vi "Read Steps From File - XML.vi"(11 "XML file path":path) -> (0 "error out":errorcluster, 3 "Sequence File Data":T1)   [LabVIEW 2011]
uses:
  HelperVIs.llb/SequenceFileData.ctl
  HelperVIs.llb/SequenceData.ctl
  HelperVIs.llb/StepGroup.ctl
  HelperVIs.llb/StepData.ctl
  HelperVIs.llb/StepProperties.ctl
  <vilib>/xml/Load XML File.vi
  <vilib>/xml/NI_XML.lvlib
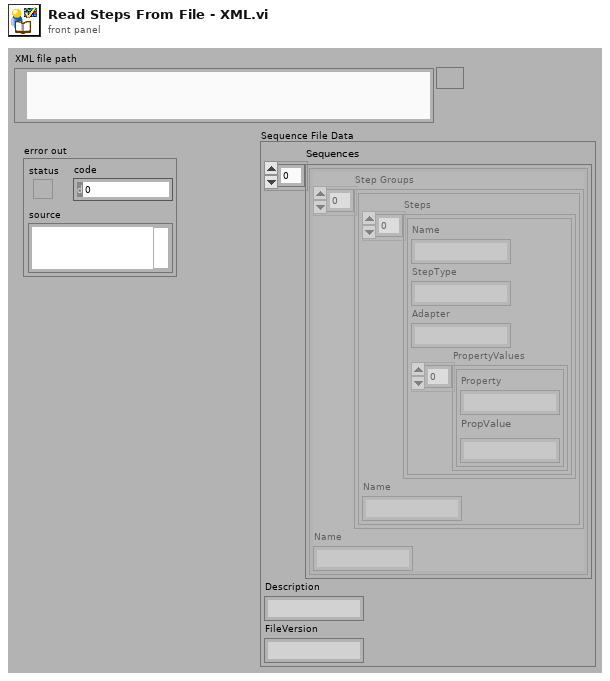
[diagram p1: front panel]
types:
  T1 = typedef "SequenceFileData.ctl" = cluster{"Sequences":T2[], "Description":string, "FileVersion":string}
  T2 = typedef "SequenceData.ctl" = cluster{"Step Groups":T3[], "Name":string}
  T3 = typedef "StepGroup.ctl" = cluster{"Steps":T4[], "Name":string}
  T4 = typedef "StepData.ctl" = cluster{"Name":string, "StepType":string, "Adapter":string, "PropertyValues":T5[]}
  T5 = typedef "StepProperties.ctl" = cluster{"Property":string, "PropValue":string}
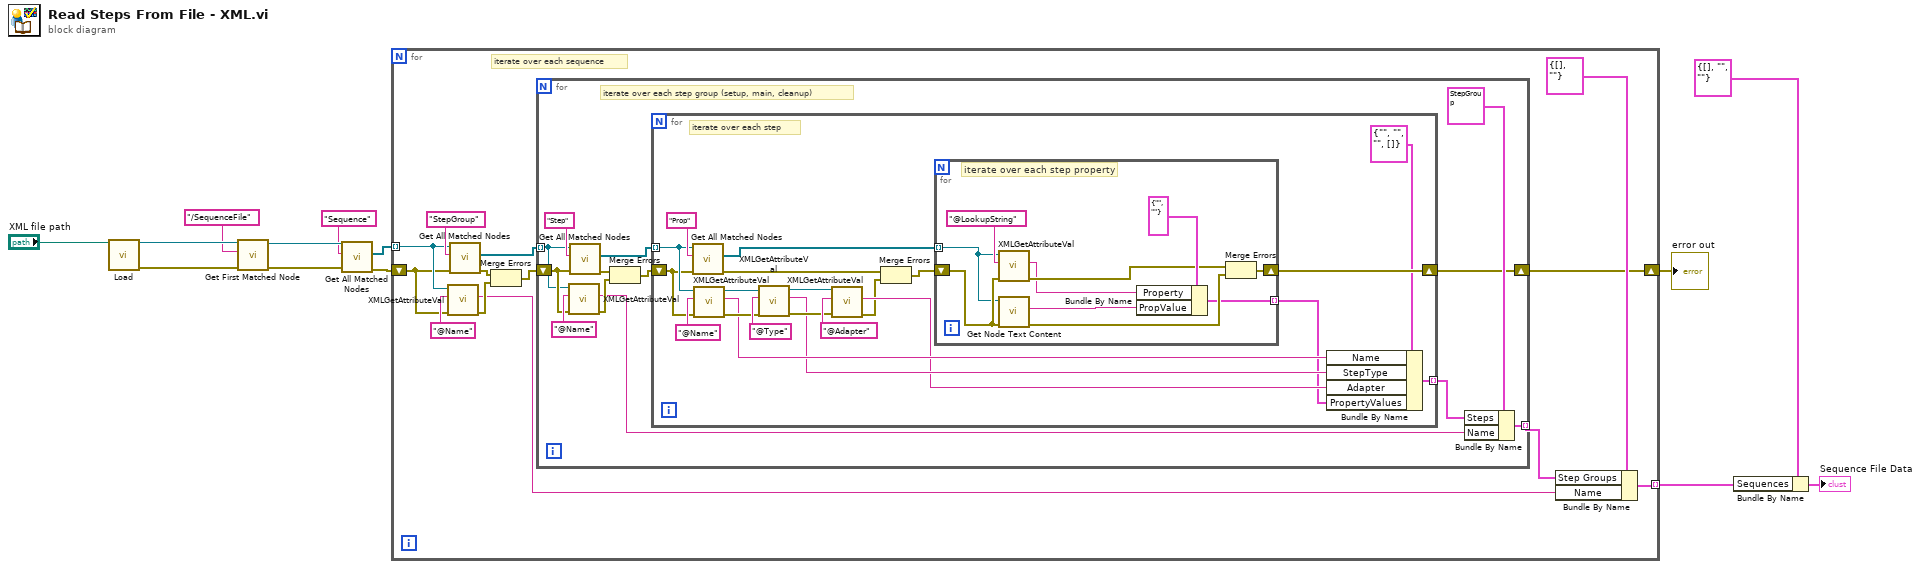
[diagram p0: block diagram]
diagram:
  n1 = call-poly <vilib>:"Load.vi"("path to XML document"="XML file path") -> ("DOM document out"=w11:refnum<k20>, "error out"=w12:errorcluster)  [unwired: 12 in, 1 out]
  n2 = call <vilib>:"Get First Matched Node.vi"("error in (no error)"=w12, "XPath expression"="/SequenceFile", "node in"=w11) -> ("error out"=w7:errorcluster, "node out"=w9:refnum<k20>)  [unwired: 6 in, 1 out]
  n3 = call <vilib>:"Get All Matched Nodes.vi"("error in (no error)"=w7, "XPath expression"="Sequence", "node in"=w9) -> ("error out"=w5:errorcluster, "node result array"=w6:refnum<k20>[])  [unwired: 6 in, 1 out]
  n4 = for {
    tunnel: w6 -> [w23] mode=indexing
    tunnel: [w17] -> w3 mode=indexing
    shift-right: [w15] -> w4
    shift-left: w5 -> [w14]
    # "iterate over each sequence"
    n5 = call "XMLGetAttributeVal.vi"("error in"=w14, "Attribute XPath"="@Name" ("XPath expression"), "Node In"=w23) -> ("error out"=w20:errorcluster, "Value"=w18:string)  [unwired: 6 in, 1 out]
    n6 = call <vilib>:"Get All Matched Nodes.vi"("error in (no error)"=w14, "XPath expression"="StepGroup", "node in"=w23) -> ("error out"=w22:errorcluster, "node result array"=w25:refnum<k20>[])  [unwired: 6 in, 1 out]
    n7 = Merge Errors(w22, w20) -> (w21:errorcluster)
    n8 = for {
      tunnel: w25 -> [w28] mode=indexing
      tunnel: [w29] -> w16 mode=indexing
      shift-right: [w27] -> w15
      shift-left: w21 -> [w34]
      # "iterate over each step group (setup, main, cleanup)"
      n9 = call "XMLGetAttributeVal.vi"("error in"=w34, "Attribute XPath"="@Name" ("XPath expression"), "Node In"=w28) -> ("error out"=w32:errorcluster, "Value"=w30:string)  [unwired: 6 in, 1 out]
      n10 = call <vilib>:"Get All Matched Nodes.vi"("error in (no error)"=w34, "XPath expression"="Step", "node in"=w28) -> ("error out"=w33:errorcluster, "node result array"=w38:refnum<k20>[])  [unwired: 6 in, 1 out]
      n11 = Merge Errors(w33, w32) -> (w31:errorcluster)
      n12 = for {
        tunnel: w38 -> [w57] mode=indexing
        tunnel: [w40] -> w36 mode=indexing
        shift-right: [w58] -> w27
        shift-left: w31 -> [w51]
        # "iterate over each step"
        n13 = call <vilib>:"Get All Matched Nodes.vi"("error in (no error)"=w51, "XPath expression"="Prop", "node in"=w57) -> ("error out"=w45:errorcluster, "node result array"=w59:refnum<k20>[])  [unwired: 6 in, 1 out]
        n14 = call "XMLGetAttributeVal.vi"("error in"=w51, "Attribute XPath"="@Name" ("XPath expression"), "Node In"=w57) -> ("error out"=w53:errorcluster, "Value"=w50:string, "Node out"=w47:refnum<k20>)  [unwired: 6 in]
        n15 = call "XMLGetAttributeVal.vi"("error in"=w53, "Attribute XPath"="@Type" ("XPath expression"), "Node In"=w47) -> ("error out"=w52:errorcluster, "Value"=w49:string, "Node out"=w46:refnum<k20>)  [unwired: 6 in]
        n16 = call "XMLGetAttributeVal.vi"("error in"=w52, "Attribute XPath"="@Adapter" ("XPath expression"), "Node In"=w46) -> ("error out"=w44:errorcluster, "Value"=w48:string)  [unwired: 6 in, 1 out]
        n17 = Merge Errors(w45, w44) -> (w43:errorcluster)
        n18 = for {
          tunnel: w59 -> [w63] mode=indexing
          tunnel: [w62] -> w42 mode=indexing
          shift-right: [w64] -> w58
          shift-left: w43 -> [w67]
          # "iterate over each step property"
          n19 = call "XMLGetAttributeVal.vi"("error in"=w67, "Attribute XPath"="@LookupString" ("XPath expression"), "Node In"=w63) -> ("error out"=w65:errorcluster, "Value"=w61:string)  [unwired: 6 in, 1 out]
          n20 = call <vilib>:"Get Node Text Content.vi"("error in (no error)"=w67, "node in"=w63) -> ("error out"=w66:errorcluster, "node text"=w70:string)  [unwired: 7 in, 1 out]
          n21 = Bundle By Name(cluster=T5 {"Property"="", "PropValue"=""} ("Property Data"), "Property"=w61, "PropValue"=w70) -> (w62:T5)
          n22 = Merge Errors(w65, w66) -> (w64:errorcluster)
        }
        n23 = Bundle By Name(cluster=T4 {"Name"="", "StepType"="", "Adapter"="", "PropertyValues"=[]} ("Step Data"), "Name"=w50, "StepType"=w49, "Adapter"=w48, "PropertyValues"=w42) -> (w40:T4)
      }
      n24 = Bundle By Name(cluster=T3 {"Steps"=[{"Name"="About", "StepType"="MessagePopup", "Adapter"="None Adapter", "PropertyValues"=[{"Property"="MessageExpr", "PropValue"="\\\"This Sequence was generated from an XML file using the TestStand API.\\\""}]}, {"Name"="", "StepType"="", "Adapter"="", "PropertyValues"=[]}], "Name"=""} ("StepGroup"), "Steps"=w36, "Name"=w30) -> (w29:T3)
    }
    n25 = Bundle By Name(cluster=T2 {"Step Groups"=[], "Name"=""} ("Sequence Data"), "Step Groups"=w16, "Name"=w18) -> (w17:T2)
  }
  "error out" <- w4
  n26 = Bundle By Name(cluster=T1 {"Sequences"=[], "Description"="", "FileVersion"=""} ("Sequence File"), "Sequences"=w3) -> (→"Sequence File Data":T1)
